vi "Create Handle Message.vi"(8 "Error In":errorcluster, 11 "Handle Message Path":path) -> (0 "Error Out":errorcluster)   [LabVIEW 2011, in "Generator.lvlib"]
uses:
  Generator.lvlib
  Type Definitions/Create Handle Message.ctl
  <vilib>/Utility/traverseref.llb/TRef TravTarget.ctl
  <vilib>/Utility/traverseref.llb/VI Scripting - Traverse.lvlib
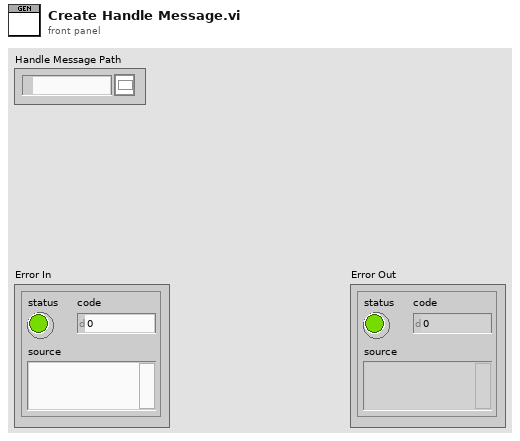
[diagram p1: front panel]
types:
  T1 = typedef "Generator.lvlib/Create Handle Message.ctl" = enum8{"Error", "Find Case Structure", "Create Type Definitions", "Create Message Handle"}
  T2 = typedef "TRef TravTarget.ctl" = enum16{"FP", "BD", "Other"}
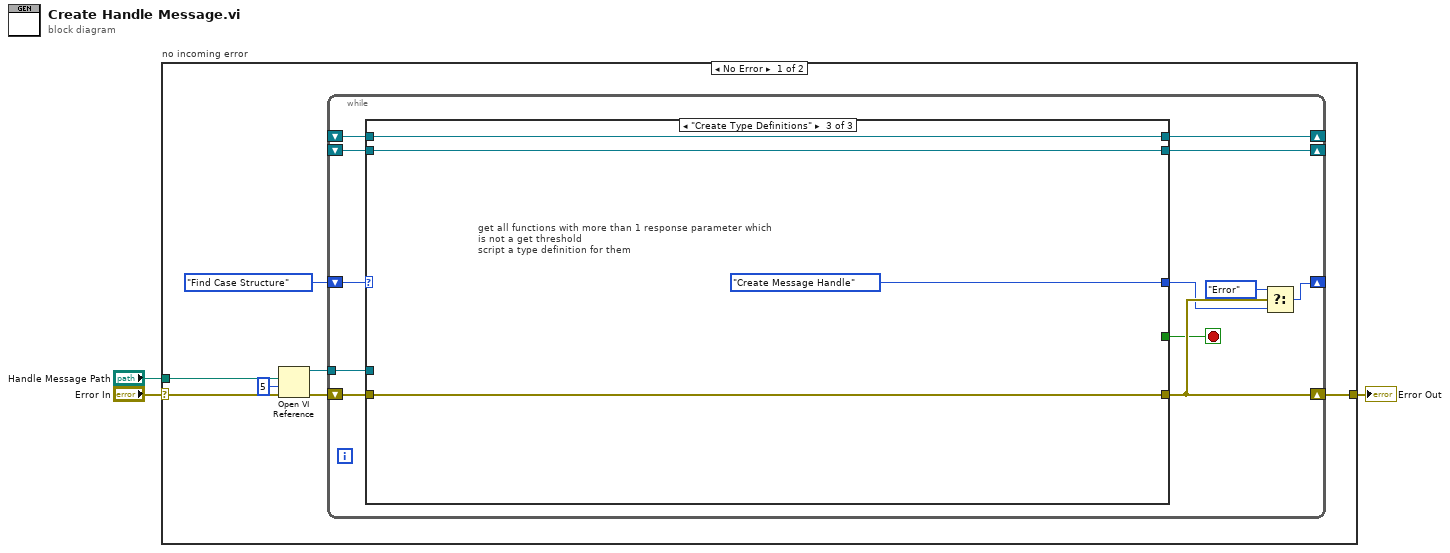
[diagram p0: block diagram]
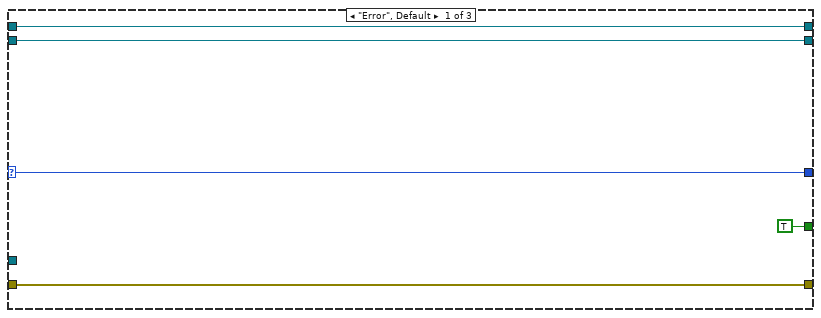
[diagram p2: hidden frame]
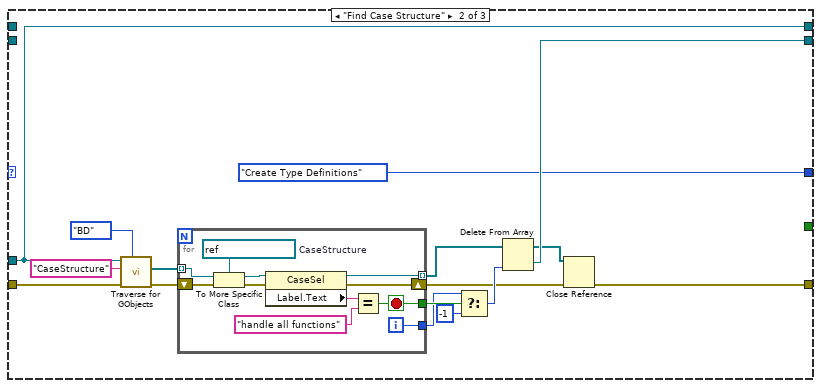
[diagram p3: hidden frame]
diagram:
  n1 = case "no incoming error" shown="No Error" "Error In" {
    selector: "Error In" -> [w10 w59]
    tunnel: [w5 w59] -> w2
    tunnel: "Handle Message Path" -> [w9 _]
    frame No Error {
      n2 = Open VI Reference(vi path=w9, options=5, error in (no error)=w10) -> (vi reference=w4:refnum<vi>, error out=w7:errorcluster)  [unwired: 3 in]
      n3 = while {
        shift-right: [w20] -> w5
        shift-left: w7 -> [w22]
        shift-right: [w18] -> _
        shift-left: Create_Handle_Message."Find Case Structure" ("State") -> [w21]
        tunnel: w4 -> [w15]
        shift-right: [w14] -> _
        shift-left: _ -> [w13]
        shift-right: [w12] -> _
        shift-left: _ -> [w11]
        stop <- w16 stop-if-true
        n4 = case shown="\"Create Type Definitions\"" w21 {
          selector: w21 -> [w26 _ _]
          tunnel: w22 -> [w27 w43 w56]
          tunnel: [w27 w29 w56] -> w20
          tunnel: [w26 Create_Handle_Message."Create Type Definitions" ("State") Create_Handle_Message."Create Message Handle" ("State")] -> w17
          tunnel: [TRUE _ _] -> w16
          tunnel: w15 -> [_ w42 _]
          tunnel: [w23 w42 w58] -> w14
          tunnel: w13 -> [w23 _ w58]
          tunnel: [w24 w32 w57] -> w12
          tunnel: w11 -> [w24 _ w57]
          frame "Error", Default {
          }
          frame "Find Case Structure" {
            n5 = call <vilib>:"Traverse for GObjects.vi"("Traverse Target"=TRef_TravTarget."BD", "error in (no error)"=w43, "Class Name"="CaseStructure", "VI Refnum"=w42) -> ("error out"=w38:errorcluster, "References"=w39:refnum<vi>[])  [unwired: 4 in, 2 out]
            n6 = for {
              tunnel: w39 -> [w53] mode=indexing
              shift-right: [w47] -> w31
              shift-left: w38 -> [w54]
              tunnel: [w46] -> w33 mode=indexing
              tunnel: [w45] -> w37
              tunnel: [w44] -> w36
              i -> [w44]
              stop <- w45 stop-if-true
              w52 = refnum<vi> refnum  # CaseStructure
              n7 = To More Specific Class(target class=w52, reference=w53, error in=w54) -> (specific class reference=w50:refnum<vi>, error out=w51:errorcluster)
              n8 = property class="CaseSel"(reference=w50, error in=w51) -> (reference out=w46:refnum<vi>, error out=w47:errorcluster, "Label.Text"=w49:string)
              n9 = Equal?(x=w49, y="handle all functions") -> (x = y?=w45:bool)
            }
            n10 = Select(t=w36, s=w37, f=-1) -> (s? t:f=w34:i32)
            n11 = Delete From Array(array=w33, index=w34) -> (deleted portion=w32:refnum<vi>, array with subset deleted=w30:refnum<vi>[])  [unwired: 1 in]
            n12 = Close Reference(reference=w30, error in (no error)=w31) -> (error out=w29:errorcluster)
          }
          frame "Create Type Definitions" {
            # "get all functions with more than 1 response parameter which\nis not a get threshold\nscript a type definition for them"
          }
        }
        n13 = Select(t=Create_Handle_Message."Error" ("State"), s=w20, f=w17) -> (s? t:f=w18:T1)
      }
    }
    frame Error {
    }
  }
  "Error Out" <- w2
